vi "ACT_Labview4task1inclass.vi"() -> ()   [LabVIEW 2016]
panel:
  out "Numeric 3":dbl
  in  "Numeric 2":dbl
  in  "Numeric":dbl
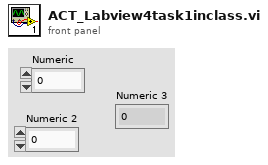
[diagram p1: front panel]
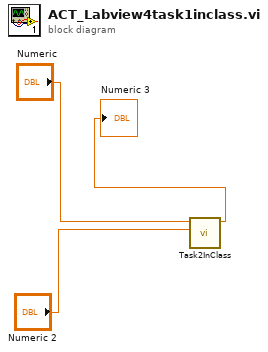
[diagram p0: block diagram]
diagram:
  n1 = call "Task2InClass.vi"("Numeric 2"="Numeric 2", "Numeric"="Numeric") -> ("Numeric 3"=→"Numeric 3":dbl)  [unwired: 9 in]
